vi "ARI Lifter Logic.vi"() -> ()   [LabVIEW 2014]
panel:
  in  "STOP":bool
  out "ARI Lift Motor":dbl
  in  "ARI Lowered Fully Switch":bool
  in  "ARI Lowered Partially Switch":bool
  in  "ARI Top Switch":bool
  in  "Motor Value":dbl min=-1.0 max=1.0 step=1.0
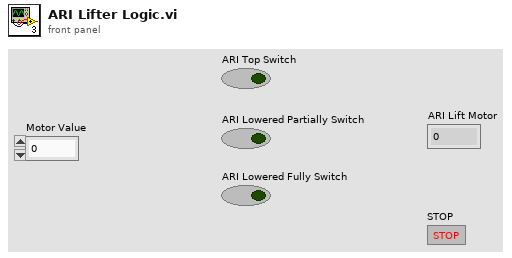
[diagram p1: front panel]
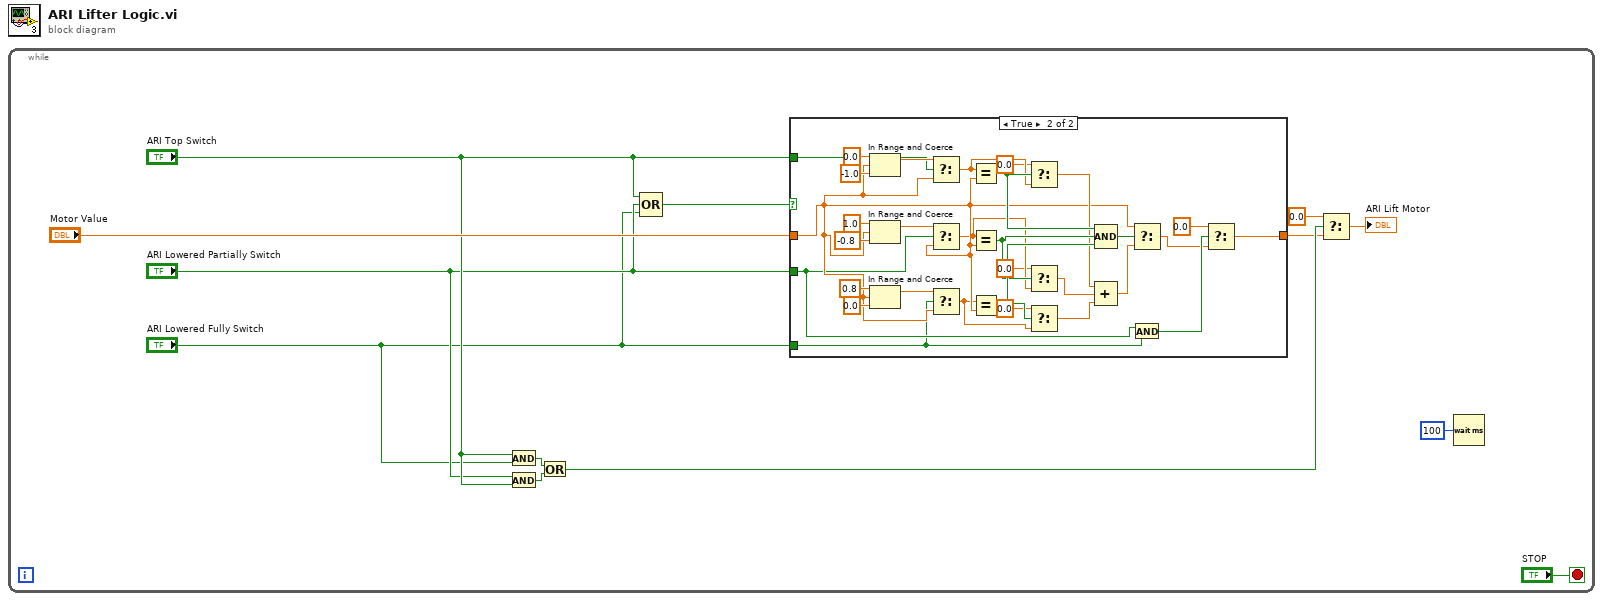
[diagram p0: block diagram]
diagram:
  n1 = while {
    stop <- "STOP" stop-if-true
    n2 = And(x="ARI Top Switch", y="ARI Lowered Fully Switch") -> (x .and. y?=w12:bool)
    n3 = And(x="ARI Lowered Partially Switch", y="ARI Top Switch") -> (x .and. y?=w11:bool)
    n4 = Or(x=w12, y=w11) -> (x .or. y?=w10:bool)
    n5 = Compound Arithmetic op=OR("ARI Top Switch", "ARI Lowered Partially Switch", "ARI Lowered Fully Switch") -> (w9:bool)
    n6 = case shown="True" w9 {
      tunnel: "ARI Lowered Fully Switch" -> [_ w19]
      tunnel: "ARI Lowered Partially Switch" -> [_ w20]
      tunnel: "Motor Value" -> [w14 w27]
      tunnel: "ARI Top Switch" -> [_ w36]
      tunnel: [w14 w15] -> w8
      frame False {
      }
      frame True {
        n7 = In Range and Coerce(upper limit=0.0, x=w27, lower limit=-1.0) -> (coerced(x)=w39:dbl)  [unwired: 1 out]
        n8 = In Range and Coerce(upper limit=1.0, x=w27, lower limit=-0.8) -> (coerced(x)=w42:dbl)  [unwired: 1 out]
        n9 = In Range and Coerce(upper limit=0.8, x=w27, lower limit=0.0) -> (coerced(x)=w45:dbl)  [unwired: 1 out]
        n10 = Select(t=w39, s=w36, f=w27) -> (s? t:f=w23:dbl)
        n11 = Select(t=w42, s=w20, f=w27) -> (s? t:f=w26:dbl)
        n12 = Select(t=w45, s=w19, f=w27) -> (s? t:f=w25:dbl)
        n13 = Equal?(x=w23, y=w27) -> (x = y?=w33:bool)
        n14 = Equal?(x=w26, y=w27) -> (x = y?=w34:bool)
        n15 = Equal?(x=w25, y=w27) -> (x = y?=w35:bool)
        n16 = Select(t=0.0, s=w33, f=w23) -> (s? t:f=w32:dbl)
        n17 = Select(t=0.0, s=w34, f=w26) -> (s? t:f=w30:dbl)
        n18 = Select(t=0.0, s=w35, f=w25) -> (s? t:f=w31:dbl)
        n19 = Compound Arithmetic op=AND(w33, w34, w35) -> (w29:bool)
        n20 = Compound Arithmetic op=ADD(w32, w30, w31) -> (w28:dbl)
        n21 = Select(t=w27, s=w29, f=w28) -> (s? t:f=w16:dbl)
        n22 = And(x=w20, y=w19) -> (x .and. y?=w18:bool)
        n23 = Select(t=0.0, s=w18, f=w16) -> (s? t:f=w15:dbl)
      }
    }
    n24 = Select(t=0.0, s=w10, f=w8) -> (s? t:f=→"ARI Lift Motor":dbl)
    n25 = Wait (ms)(milliseconds to wait=u32 100) -> ()  [unwired: 1 out]
  }
